vi "Set Custom Device Dependent File Properties.vi"(7 "Format Settings":T1, 8 "error in (no error)":errorcluster, 10 "Dependent Files":T2[](array[typedef]) {"Type" items=["Absolute", "ToBase", "ToCommonDocDir", "ToApplicationDataDir"]}, 11 "BaseNodeType":refnum<k24>) -> (0 "error out":errorcluster, 3 "BaseNodeType out":refnum<k24>)   [LabVIEW 2020, in "VeriStand SLSC Scripting.lvlib"]
uses:
  VeriStand SLSC Scripting.lvlib
  Controls/Dependent File Information.ctl
  <vilib>/NI VeriStand/Custom Device API/Custom Device Supported Target.ctl
  NationalInstruments.VeriStand.SystemStorage
  <vilib>/NI VeriStand/Custom Device API/Custom Device API.lvlib
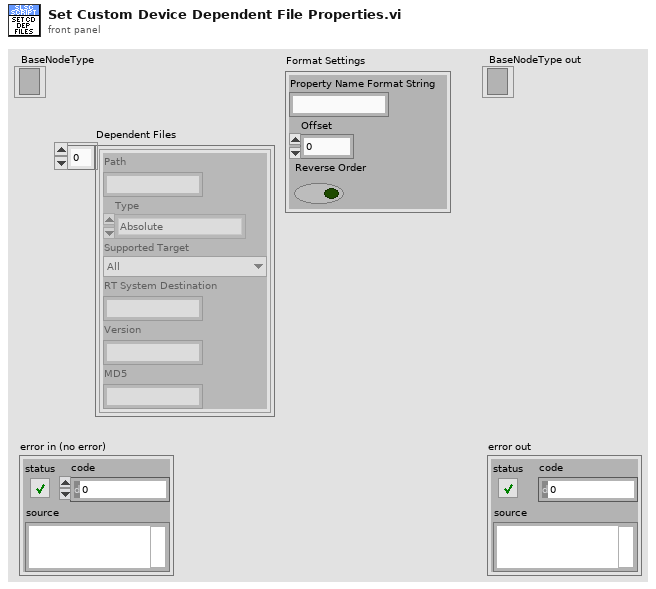
[diagram p1: front panel]
types:
  T1 = cluster{"Property Name Format String":string, "Offset":i32, "Reverse Order":bool}
  T2 = typedef "VeriStand SLSC Scripting.lvlib/Dependent File Information.ctl" = cluster{"Path":string, "Type":i32, "Supported Target":T3, "RT System Destination":string, "Version":string, "MD5":string}
  T3 = typedef "Custom Device API.lvlib/Custom Device Supported Target.ctl" = enum16{"All", "PharLap", "VxWorks", "Windows", "Linux_32_ARM", "Linux_x64", "PharLap & Windows", "PharLap & VxWorks", "VxWorks & Windows"}
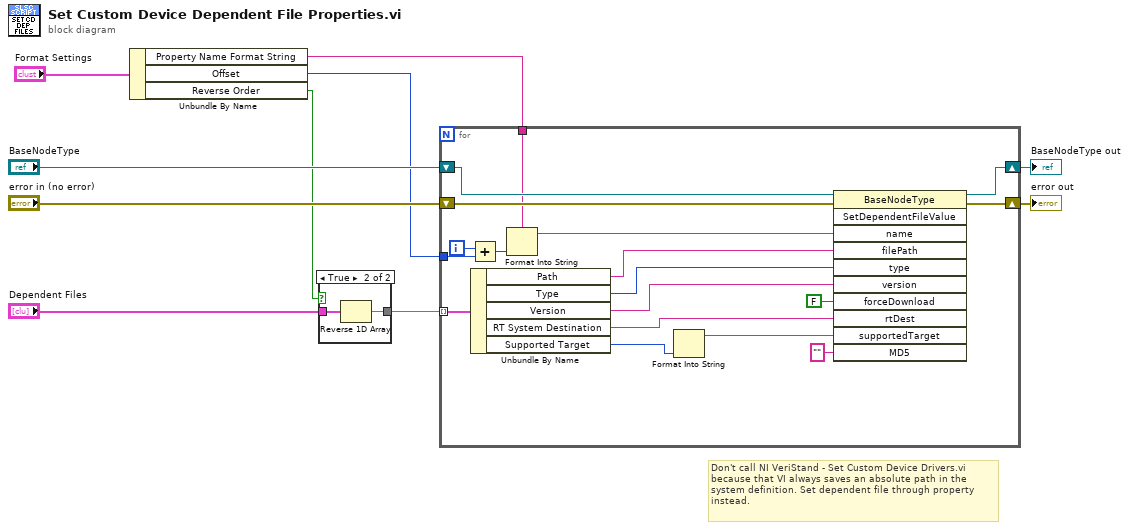
[diagram p0: block diagram]
diagram:
  # "Don't call NI VeriStand - Set Custom Device Drivers.vi\nbecause that VI always saves an absolute path in the\nsystem definition. Set dependent file through property\ninstead."
  n1 = Unbundle By Name("Format Settings") -> ("Property Name Format String"=w5:string, "Offset"=w4:i32, "Reverse Order"=w2:bool)
  n2 = case shown="True" w2 {
    tunnel: "Dependent Files" -> [w11 w13]
    tunnel: [w11 w12] -> w1
    frame False {
    }
    frame True {
      n3 = Reverse 1D Array(array=w13) -> (reversed array=w12:T2[])
    }
  }
  n4 = for {
    shift-right: [w28] -> w8
    shift-left: "error in (no error)" -> [w31]
    shift-right: [w29] -> w7
    shift-left: "BaseNodeType" -> [w30]
    tunnel: w1 -> [w27] mode=indexing
    tunnel: w5 -> [w17]
    tunnel: w4 -> [w14]
    i -> [w16]
    n5 = Add(x=w16, y=w14) -> (x+y=w15:i32)
    n6 = Unbundle By Name(w27) -> ("Path"=w25:string, "Type"=w24:i32, "Version"=w23:string, "RT System Destination"=w21:string, "Supported Target"=w19:T3)
    n7 = Format Into String(format string=w17, w15) -> (resulting string=w26:string)  [unwired: 2 in, 1 out]
    n8 = Format Into String(w19) -> (resulting string=w18:string)  [unwired: 3 in, 1 out]
    n9 = invoke class="BaseNodeType" method="SetDependentFileValue"(reference=w30, error in=w31, "name"=w26, "filePath"=w25, "type"=w24, "version"=w23, "forceDownload"=FALSE, "rtDest"=w21, "supportedTarget"=w18, "MD5"="") -> (reference out=w29:refnum<k24>, error out=w28:errorcluster)  [unwired: 1 in, 9 out]
  }
  "error out" <- w8
  "BaseNodeType out" <- w7
